vi "MyrioProject.vi"() -> ()   [LabVIEW 2018]
doc: "The myRIO Project template acquires acceleration data from the onboard accelerometer and displays the changes of acceleration values in a waveform chart."
uses:
  <vilib>/Platform/TimedLoop/XDataNode/timing_clust.ctl
  <vilib>/Platform/TimedLoop/XDataNode/nitl_modes.ctl
  <vilib>/Platform/TimedLoop/XDataNode/wakeup.ctl
  <vilib>/myRIO/Common/Instrument Driver Framework/myRIO v1.0/Encoder/typedefs/Encoder Signal Mode.ctl
  <vilib>/myRIO/Instrument Drivers/Onboard IO/PWM/typedefs/PWM Reference.ctl
  <vilib>/myRIO/Common/Instrument Driver Framework/Utilities/typedefs/myRIO Generic Hardware Reference.ctl
  <vilib>/myRIO/Common/Instrument Driver Framework/Utilities/typedefs/Hardware Version Enum.ctl
  <vilib>/myRIO/Common/Instrument Driver Framework/Utilities/typedefs/myRIO v1.0 Reference.ctl
  <vilib>/myRIO/Common/Instrument Driver Framework/Utilities/typedefs/Generic FPGA Reference.ctl
  <vilib>/myRIO/Common/Instrument Driver Framework/myRIO v1.0/PWM/typedefs/PWM Channels Enum.ctl
  <vilib>/myRIO/Instrument Drivers/Onboard IO/PWM/typedefs/PWM Configuration.ctl
  <vilib>/userdefined/High Color/nirio_resource_hc.ctl
  <vilib>/myRIO/Common/Instrument Driver Framework/myRIO v1.0/Encoder/typedefs/Encoder Configuration v1.0.ctl
  <vilib>/myRIO/Instrument Drivers/Onboard IO/Encoder/typedefs/Encoder Reference.ctl
  <vilib>/myRIO/Common/Instrument Driver Framework/myRIO v1.0/Encoder/typedefs/Encoder Channels Enum.ctl
  <vilib>/myRIO/Instrument Drivers/Onboard IO/DIO/typedefs/DIO Reference.ctl
  <vilib>/myRIO/Common/Instrument Driver Framework/myRIO v1.0/DIO/typedefs/DIO Channels List.ctl
  <vilib>/myRIO/Common/Instrument Driver Framework/myRIO v1.0/DIO/typedefs/DIO Channels Enum.ctl
  <vilib>/myRIO/Instrument Drivers/Onboard IO/AI/typedefs/AI Reference.ctl
  <vilib>/myRIO/Common/Instrument Driver Framework/myRIO v1.0/AI/typedefs/AI Channels List.ctl
  <vilib>/myRIO/Common/Instrument Driver Framework/myRIO v1.0/AI/typedefs/AI Channels Enum.ctl
  <vilib>/myRIO/Common/Instrument Driver Framework/Utilities/typedefs/Analog Scaling Constants List.ctl
  <vilib>/myRIO/Common/Instrument Driver Framework/Utilities/typedefs/Analog Scaling Constants.ctl
  <vilib>/myRIO/Common/Instrument Driver Framework/myRIO v1.0/PWM/vis/myRIO v1.1 Open PWM.vi
  <vilib>/myRIO/Common/Instrument Driver Framework/myRIO v1.0/Encoder/vis/myRIO v1.1 Open Encoder.vi
  <vilib>/myRIO/Common/Instrument Driver Framework/Utilities/vis/Is FPGA Ref Available.vi
  <vilib>/myRIO/Common/Instrument Driver Framework/myRIO v1.0/AI/vis/myRIO v1.1 Open AI.vi
  <vilib>/myRIO/Common/Instrument Driver Framework/myRIO v1.0/DIO/vis/myRIO v1.1 Open DIO.vi
  <vilib>/myRIO/Instrument Drivers/Onboard IO/PWM/vis/Set Duty Cycle and Frequency.vi
  <vilib>/myRIO/Instrument Drivers/Onboard IO/DIO/vis/Write.vi
  <vilib>/myRIO/Common/Instrument Driver Framework/Utilities/vis/Validate Channels.vi
  <vilib>/myRIO/Common/Instrument Driver Framework/myRIO v1.0/PWM/vis/myRIO v1.0 Reserve PWM.vi
  <vilib>/myRIO/Common/Instrument Driver Framework/myRIO v1.0/Encoder/vis/myRIO v1.0 Reserve Encoder.vi
  <vilib>/myRIO/Common/Instrument Driver Framework/myRIO v1.0/AI/vis/myRIO v1.0 Reserve AI.vi
  <vilib>/myRIO/Common/Instrument Driver Framework/myRIO v1.0/DIO/vis/myRIO v1.0 Reserve DIO.vi
  <vilib>/myRIO/Common/Instrument Driver Framework/myRIO v1.0/Encoder/vis/myRIO v1.0 Close Encoder.vi
  <vilib>/myRIO/Common/Instrument Driver Framework/myRIO v1.0/PWM/vis/myRIO v1.0 Close PWM.vi
  <vilib>/myRIO/Common/Instrument Driver Framework/myRIO v1.0/PWM/vis/myRIO v1.0 Build MUX Configuration PWM.vi
  <vilib>/myRIO/Common/Instrument Driver Framework/myRIO v1.0/Resource Manager/vis/myRIO v1.0 Reserve Channel List.vi
  <vilib>/myRIO/Common/Instrument Driver Framework/myRIO v1.0/Encoder/vis/myRIO v1.0 Build MUX Configuration Encoder.vi
  <vilib>/myRIO/Common/Instrument Driver Framework/myRIO v1.0/AI/vis/myRIO v1.0 Build MUX Configuration AI.vi
  <vilib>/myRIO/Common/Instrument Driver Framework/myRIO v1.0/DIO/vis/myRIO v1.0 Build MUX Configuration DIO.vi
  <vilib>/myRIO/Common/Instrument Driver Framework/myRIO v1.0/Encoder/vis/myRIO v1.0 Unreserve Encoder.vi
  <vilib>/myRIO/Common/Instrument Driver Framework/myRIO v1.0/PWM/vis/myRIO v1.0 Unreserve PWM.vi
  <vilib>/myRIO/Common/Instrument Driver Framework/myRIO v1.0/Resource Manager/vis/myRIO v1.0 Create Configuration List.vi
  <vilib>/myRIO/Common/Instrument Driver Framework/myRIO v1.0/Resource Manager/vis/myRIO v1.0 Reserve Channel.vi
  <vilib>/myRIO/Common/Instrument Driver Framework/myRIO v1.0/Resource Manager/vis/myRIO v1.0 Unreserve Channel.vi
  <vilib>/myRIO/Common/Instrument Driver Framework/myRIO v1.0/Resource Manager/vis/myRIO v1.0 Unreserve Channel List.vi
  <vilib>/myRIO/Common/Instrument Driver Framework/myRIO v1.0/Resource Manager/vis/myRIO v1.0 Build Mutex Name.vi
  <vilib>/Utility/VariantDataType/GetNumericInfo.vi
  <vilib>/Utility/error.llb/Error Cluster From Error Code.vi
  <vilib>/myRIO/Common/Instrument Driver Framework/myRIO v1.0/myRIO v1.1 Open.vi
  <vilib>/myRIO/Common/Instrument Driver Framework/Utilities/vis/IO Manager.vi
  <vilib>/myRIO/Common/Instrument Driver Framework/Utilities/vis/Configuration Manager.vi
  <vilib>/myRIO/Common/Instrument Driver Framework/myRIO v1.0/Resource Manager/vis/myRIO v1.0 Configure IO.vi
  <vilib>/myRIO/Common/Instrument Driver Framework/myRIO v1.0/myRIO v1.0 Close.vi
  <vilib>/myRIO/Common/Instrument Driver Framework/myRIO v1.0/PWM/vis/myRIO v1.0 Write PWM.vi
  <vilib>/myRIO/Common/Instrument Driver Framework/myRIO v1.0/Encoder/vis/myRIO v1.0 Configure Encoder.vi
  <vilib>/myRIO/Common/Instrument Driver Framework/myRIO v1.0/Encoder/vis/myRIO v1.0 Enable Encoder.vi
  <vilib>/myRIO/Common/Instrument Driver Framework/myRIO v1.0/DIO/vis/myRIO v1.0 Read DIO.vi
  <vilib>/myRIO/Common/Instrument Driver Framework/myRIO v1.0/AI/vis/myRIO v1.0 Get Scaling Constants AI.vi
  <vilib>/myRIO/Common/Instrument Driver Framework/myRIO v1.0/AI/vis/myRIO v1.0 Read AI.vi
  <vilib>/myRIO/Common/Instrument Driver Framework/myRIO v1.0/Encoder/vis/myRIO v1.0 Read Encoder.vi
  <vilib>/myRIO/Common/Instrument Driver Framework/myRIO v1.0/DIO/vis/myRIO v1.0 Write DIO.vi
  <vilib>/myRIO/Common/Instrument Driver Framework/myRIO v1.0/Encoder/vis/myRIO v1.0 Shutdown Encoder.vi
  <vilib>/myRIO/Common/Instrument Driver Framework/myRIO v1.0/PWM/vis/myRIO v1.0 Shutdown PWM.vi
  <vilib>/platform/TimedLoop/XDataNode/XDataNode.xnode
  <vilib>/myRIO/Instrument Drivers/Onboard IO/PWM/vis/myRIO PWM Open.xnode
  <vilib>/myRIO/Instrument Drivers/Onboard IO/Encoder/vis/myRIO Encoder Open.xnode
  <vilib>/myRIO/Express VI/Onboard IO/PWM/PWM Express VI.xnode
  <vilib>/myRIO/Express VI/Onboard Devices/Button/Button Express VI.xnode
  <vilib>/myRIO/Instrument Drivers/Onboard IO/DIO/vis/myRIO DIO Open.xnode
  <vilib>/myRIO/Express VI/Onboard IO/AI/AI Express VI.xnode
  <vilib>/myRIO/Instrument Drivers/Onboard IO/AI/vis/myRIO AI Open.xnode
  <vilib>/myRIO/Express VI/Onboard IO/DO/DO Express VI.xnode
  <vilib>/Platform/TimedLoop/XDataNode/XDNodeRunTimeDep.lvlib
  <vilib>/myRIO/Instrument Drivers/Onboard IO/Encoder/Encoder.lvlib
  <vilib>/myRIO/Instrument Drivers/Onboard IO/PWM/PWM.lvlib
  <vilib>/myRIO/Instrument Drivers/Onboard IO/DIO/DIO.lvlib
  <vilib>/myRIO/Instrument Drivers/Onboard IO/AI/AI.lvlib
panel:
  out "Waveform Chart":dbl(graph)
  out "Numeric Control":dbl
  out "data":dbl
  out "Double 2":dbl
  out "Double":dbl
  out "sensor2 (A/AI2 (Pin 7))":dbl
  out "sensor1":dbl
  out "stallRojo (A/AI0 (Pin 3))":dbl
  out "stallBlanco (A/AI1 (Pin 5))":dbl
  in  "MANUAL 2":bool
  in  "Stop Button":bool
  in  "Start":bool
  out "element":dbl
  out "element 2":dbl
  out "subarray 2":dbl[][](array[numeric])
  out "subarray":dbl[][](array[numeric])
  out "vectores":dbl[][][](array[numeric])
  in  "saturacion":dbl=0.3
  in  "Duty Cycle 2":dbl(slide)=0.5 scale=0.05..0.1
  in  "Duty Cycle":dbl(slide)=0.5 scale=0.05..0.1
  in  "Reset Counter 2":bool
  in  "Reset Counter":bool
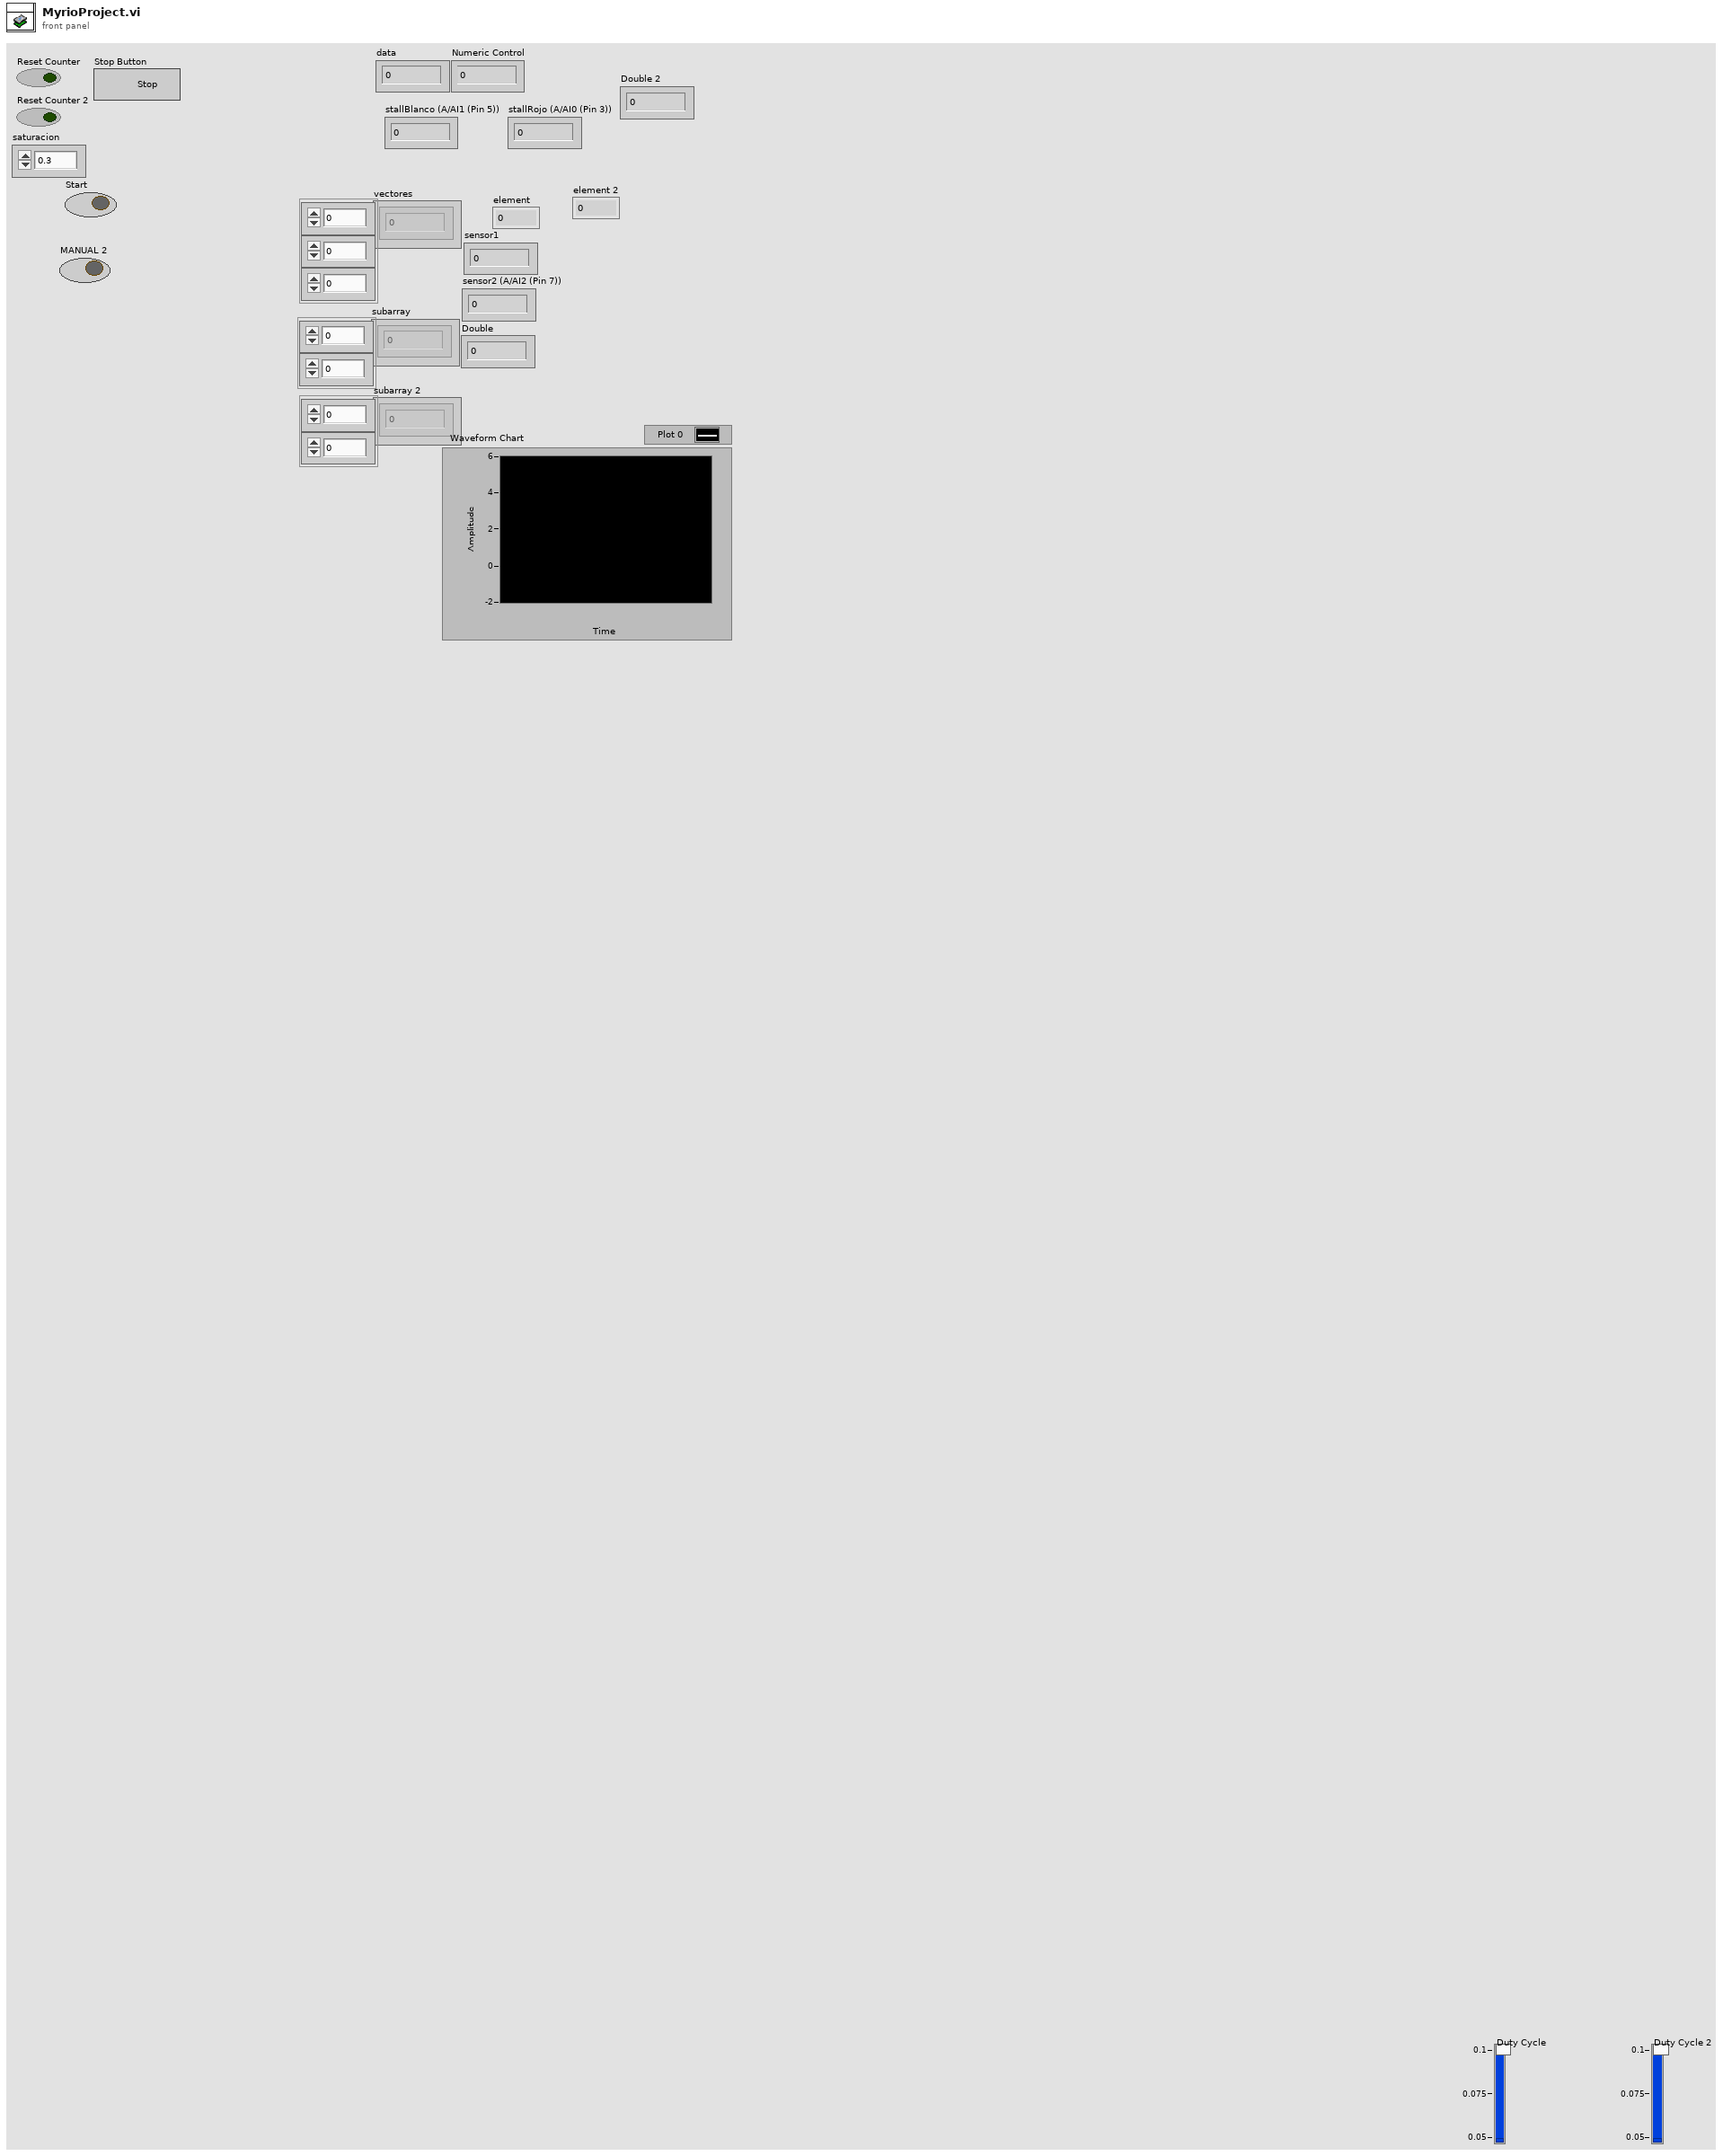
[diagram p1: front panel]
types:
  T1 = enum16{"normal", "grande-Sensor", "grande home", "peque-sensor", "peque- home", "peque-reset"}
  T2 = typedef "Encoder Signal Mode.ctl" = enum16{"Quadrature phase signal", "Step and direction signal"}
  T3 = typedef "PWM.lvlib/PWM Reference.ctl" = cluster{"myRIO Reference":T4, "PWM Channels Enum":T8, "PWM Configuration":T9}
  T4 = typedef "myRIO Generic Hardware Reference.ctl" = cluster{"myRIO Model":T5, "myRIO Hardware Reference":T6}
  T5 = typedef "Hardware Version Enum.ctl" = enum16{"Unknown", "myRIO-1900", "myRIO-1950", "roboRIO", "NI ELVIS RIO CM", "ELVIS III"}
  T6 = typedef "myRIO v1.0 Reference.ctl" = cluster{"Generic FPGA Reference":T7, "Allow multiple opens":bool}
  T7 = typedef "Generic FPGA Reference.ctl" = refnum<k20>
  T8 = typedef "PWM Channels Enum.ctl" = enum16{"Not Connected", "C/PWM0", "C/PWM1", "A/PWM0", "A/PWM1", "A/PWM2", "A/PWM3", "A/PWM4", "A/PWM5", "A/PWM6", "A/PWM7", "A/PWM8", "A/PWM9", "A/PWM10", "A/PWM11", "A/PWM12", "A/PWM13", "A/PWM14", "A/PWM15", "A/PWM16", "A/PWM17", "A/PWM18", "A/PWM19", "B/PWM0", "B/PWM1", "B/PWM2", "B/PWM3", "B/PWM4", "B/PWM5", "B/PWM6", "B/PWM7", "B/PWM8", "B/PWM9", "B/PWM10", "B/PWM11", "B/PWM12", "B/PWM13", "B/PWM14", "B/PWM15", "B/PWM16", "B/PWM17", "B/PWM18", "B/PWM19", "PWM/PWM0", "PWM/PWM1", "PWM/PWM2", "PWM/PWM3", "PWM/PWM4", "PWM/PWM5", "PWM/PWM6", "PWM/PWM7", "PWM/PWM8", "PWM/PWM9"}
  T9 = typedef "PWM.lvlib/PWM Configuration.ctl" = cluster{"Frequency":dbl, "Duty Cycle":dbl}
  T10 = typedef "Encoder.lvlib/Encoder Reference.ctl" = cluster{"myRIO Reference":T4, "Encoder Channels Enum":T11}
  T11 = typedef "Encoder Channels Enum.ctl" = enum16{"Not Connected", "C/ENC0", "C/ENC1", "A/ENC", "A/ENC0", "A/ENC1", "A/ENC2", "A/ENC3", "A/ENC4", "A/ENC5", "A/ENC6", "A/ENC7", "A/ENC8", "A/ENC9", "B/ENC", "B/ENC0", "B/ENC1", "B/ENC2", "B/ENC3", "B/ENC4", "B/ENC5", "B/ENC6", "B/ENC7", "B/ENC8", "B/ENC9", "DIO/ENC0", "DIO/ENC1", "DIO/ENC2", "DIO/ENC3", "DIO/ENC4"}
  T12 = typedef "XDNodeRunTimeDep.lvlib/timing_clust.ctl" = cluster{"Expected End [f-1]":u64, "Actual End [f-1]":u64, "Finished Late? [f-1]":bool, "Expected End [i-1]":u64, "Actual End [i-1]":u64, "Finished Late? [i-1]":bool, "Expected Start [i]":u64, "Actual Start [i]":u64, "Expected Start [f]":u64, "Actual Start [f]":u64, "Source Name":string, "Structure Name":string, "Period":i64, "Deadline":i64, "Offset":i64, "Start":i64, "Priority":i32, "Timeout":i32, "Mode":T13, "Wakeup Reason":T14, "Error":errorcluster, "Source Type":string, "Secondary Source Type":string, "Global End Time":u64, "Global Start Time":u64, "Frame Duration":u64, "Iteration Duration":u64, "Assigned CPU":i32, "I/O Scan Engine Mode":u32}
  T13 = typedef "XDNodeRunTimeDep.lvlib/nitl_modes.ctl" = enum32{"No Change", "Process missed periods, maintain original phase", "Discard missed periods, maintain original phase", "Process missed periods, ignore original phase", "Discard missed periods, ignore original phase"}
  T14 = typedef "XDNodeRunTimeDep.lvlib/wakeup.ctl" = enum32{"Normal", "Aborted", "Asynchronous wakeup", "Timing source error", "Timed loop error", "Timeout"}
  T15 = typedef "nirio_resource_hc.ctl" = tag
  T16 = typedef "AI.lvlib/AI Reference.ctl" = cluster{"myRIO Reference":T4, "AI Channels List":T17, "AI Scaling Constants List":T19}
  T17 = typedef "AI Channels List.ctl" = T18[]
  T18 = typedef "AI Channels Enum.ctl" = enum16{"Not Connected", "AudioIn/Left", "AudioIn/Right", "C/AI0", "C/AI1", "A/AI0", "A/AI1", "A/AI2", "A/AI3", "A/AI4", "A/AI5", "A/AI6", "A/AI7", "B/AI0", "B/AI1", "B/AI2", "B/AI3", "B/AI4", "B/AI5", "B/AI6", "B/AI7", "AI/AI0", "AI/AI1", "AI/AI2", "AI/AI3", "A/AI0 (DIFF)", "A/AI1 (DIFF)", "A/AI2 (DIFF)", "A/AI3 (DIFF)", "B/AI0 (DIFF)", "B/AI1 (DIFF)", "B/AI2 (DIFF)", "B/AI3 (DIFF)"}
  T19 = typedef "Analog Scaling Constants List.ctl" = T20[]
  T20 = typedef "Analog Scaling Constants.ctl" = cluster{"LSB Weight (Volts)":dbl, "Offset (Volts)":dbl, "Signed?":bool}
  T21 = typedef "DIO.lvlib/DIO Reference.ctl" = cluster{"myRIO Reference":T4, "DIO Channels List":T22}
  T22 = typedef "DIO Channels List.ctl" = T23[]
  T23 = typedef "DIO Channels Enum.ctl" = enum16{"Not Connected", "C/DIO0", "C/DIO1", "C/DIO2", "C/DIO3", "C/DIO4", "C/DIO5", "C/DIO6", "C/DIO7", "A/DIO0", "A/DIO1", "A/DIO2", "A/DIO3", "A/DIO4", "A/DIO5", "A/DIO6", "A/DIO7", "A/DIO8", "A/DIO9", "A/DIO10", "A/DIO11", "A/DIO12", "A/DIO13", "A/DIO14", "A/DIO15", "A/DIO16", "A/DIO17", "A/DIO18", "A/DIO19", "B/DIO0", "B/DIO1", "B/DIO2", "B/DIO3", "B/DIO4", "B/DIO5", "B/DIO6", "B/DIO7", "B/DIO8", "B/DIO9", "B/DIO10", "B/DIO11", "B/DIO12", "B/DIO13", "B/DIO14", "B/DIO15", "B/DIO16", "B/DIO17", "B/DIO18", "B/DIO19", "LED0", "LED1", "LED2", "LED3", "Button0", "DIO/DIO0", "DIO/DIO1", "DIO/DIO2", "DIO/DIO3", "DIO/DIO4", "DIO/DIO5", "DIO/DIO6", "DIO/DIO7", "DIO/DIO8", "DIO/DIO9", "SPI/CS0", "SPI/CS1", "SPI/CS2", "SPI/CS3", "LED RADIO (Green)", "LED RADIO (Red)", "LED COMM (Green)", "LED COMM (Red)", "LED MODE (Green)", "LED MODE (Red)"}
  T24 = cluster{dbl, dbl, "Counter Value":i32, "seconds since 1Jan1904":timestamp, dbl, dbl, dbl}
  T25 = cluster{"Double":dbl, "dbl Scaled Value":dbl, "Output":dbl, "seconds since 1Jan1904":timestamp, dbl, dbl, dbl}
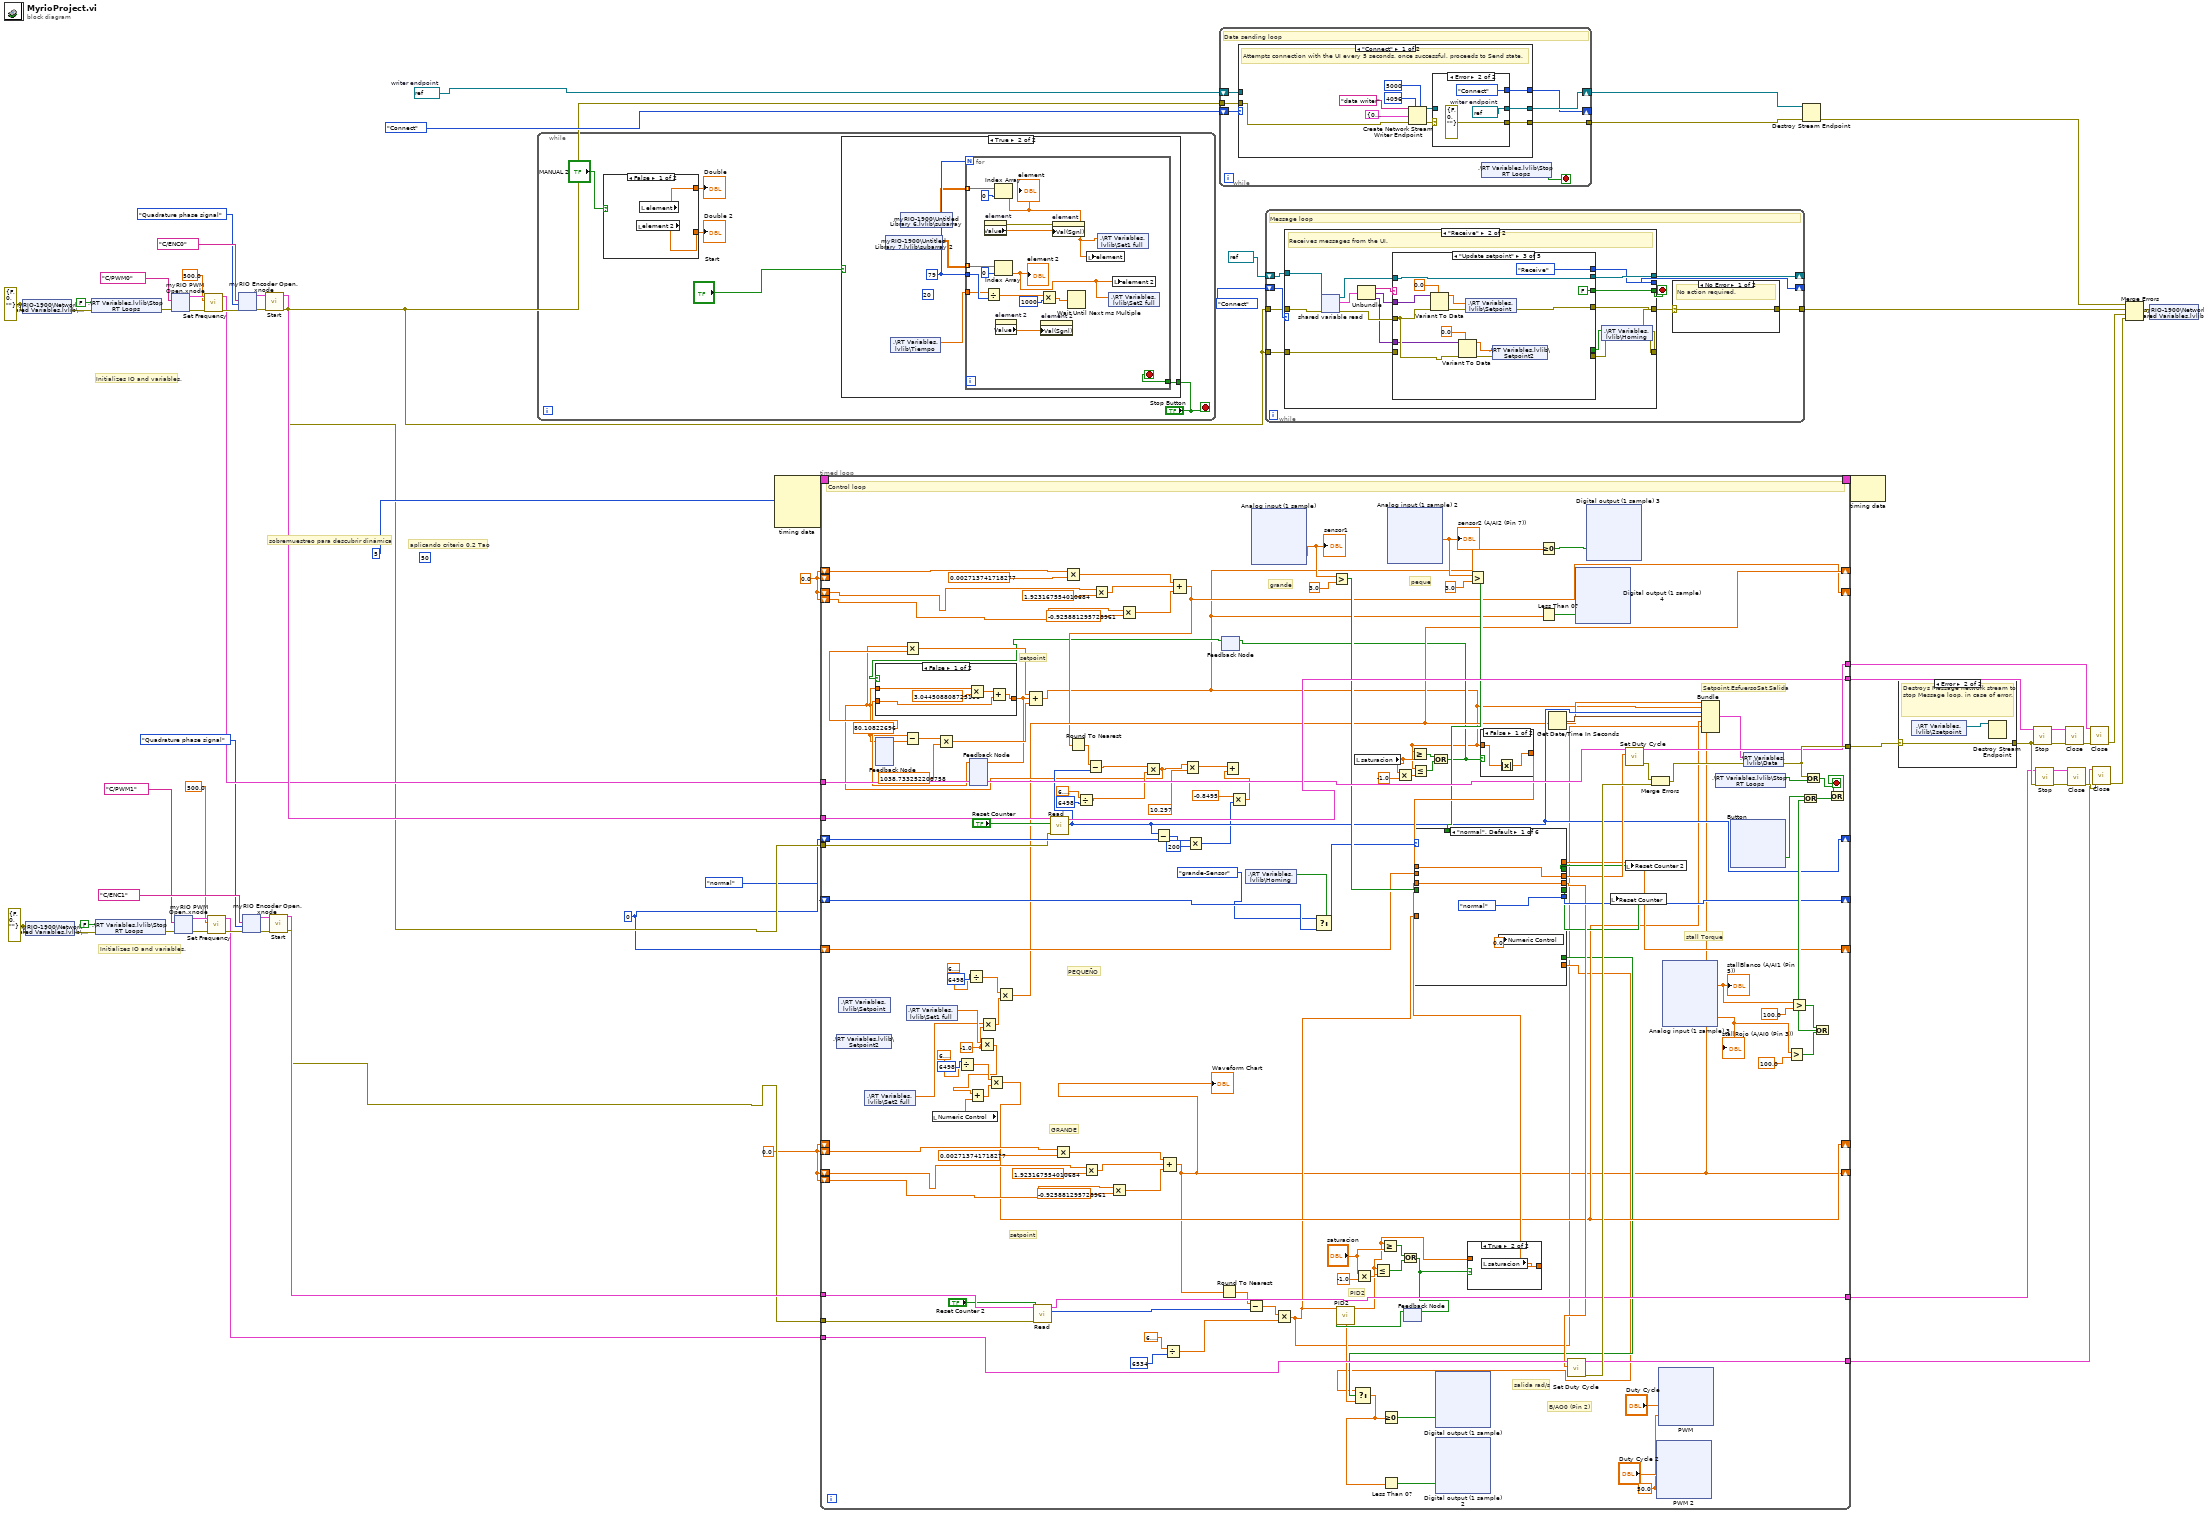
[diagram p0: block diagram]
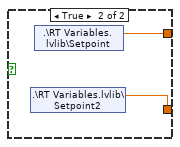
[diagram p2: hidden frame]
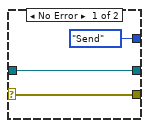
[diagram p5: hidden frame]
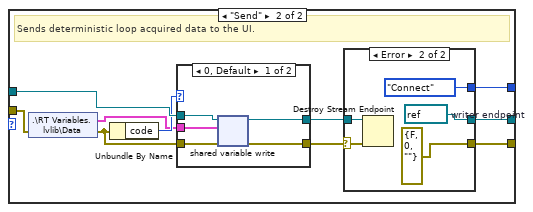
[diagram p6: hidden frame]
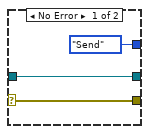
[diagram p7: hidden frame]
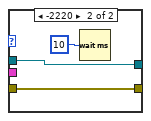
[diagram p8: hidden frame]
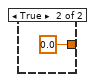
[diagram p9: hidden frame]
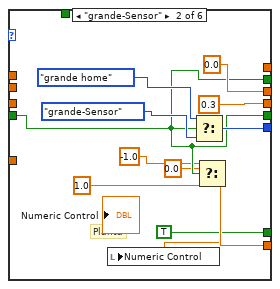
[diagram p10: hidden frame]
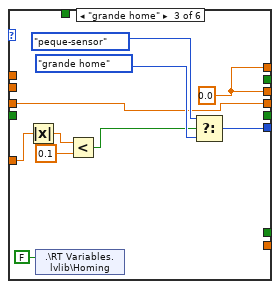
[diagram p11: hidden frame]
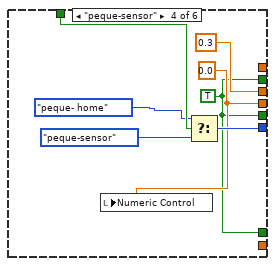
[diagram p12: hidden frame]
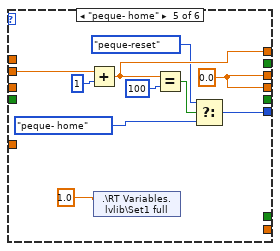
[diagram p13: hidden frame]
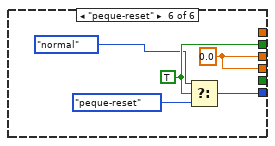
[diagram p14: hidden frame]
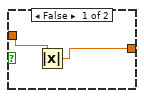
[diagram p15: hidden frame]
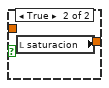
[diagram p16: hidden frame]
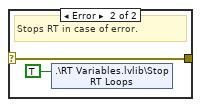
[diagram p17: hidden frame]
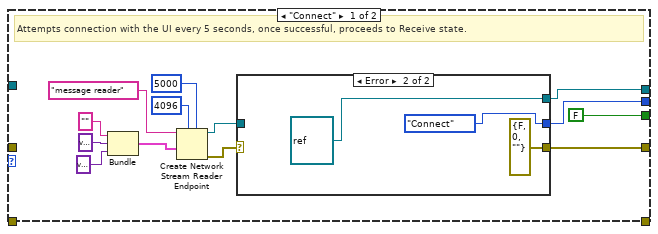
[diagram p18: hidden frame]
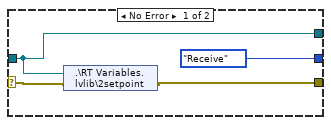
[diagram p19: hidden frame]
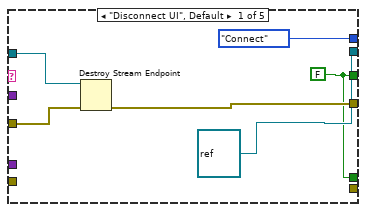
[diagram p20: hidden frame]
diagram:
  w2 = 0.0
  w3 = 0.0
  w4 = 0
  (unwired) 50
  w16 = refnum<k21> refnum  # writer endpoint
  w29 = errorcluster {"status"=FALSE, "code"=0, "source"=""} ("error IO")
  w51 = errorcluster {"status"=FALSE, "code"=0, "source"=""} ("error IO")
  # "aplicando criterio 0.2 Tao"
  # "sobremuestreo para descubrir dinámica"
  # "Initializes IO and variables."
  # "Initializes IO and variables."
  n1 = shared-variable "myRIO-1900\\Network Shared Variables.lvlib\\error IO"(w51, error in=w51) -> (error out=w52:errorcluster)
  n2 = shared-variable "myRIO-1900\\Network Shared Variables.lvlib\\error IO"(w29, error in=w29) -> (error out=w30:errorcluster)
  n3 = shared-variable ".\\RT Variables.lvlib\\Stop RT Loops"(FALSE ("Stop RT Loops"), error in=w52) -> (error out=w39:errorcluster)
  n4 = shared-variable ".\\RT Variables.lvlib\\Stop RT Loops"(FALSE ("Stop RT Loops"), error in=w30) -> (error out=w22:errorcluster)
  n5 = xnode "myRIO PWM Open.xnode"("error in (no error)"=w39, "Channel Name"=tag "C/PWM0") -> ("error out"=w41:errorcluster, "PWM Ref Out"=w40:T3)  [unwired: 1 in]
  n6 = xnode "myRIO PWM Open.xnode"("error in (no error)"=w22, "Channel Name"=tag "C/PWM1") -> ("error out"=w24:errorcluster, "PWM Ref Out"=w23:T3)  [unwired: 1 in]
  n7 = call <vilib>:"Set Frequency.vi"("error in (no error)"=w41, "Frequency [Hz]"=500.0, "PWM Ref In"=w40) -> ("error out"=w38:errorcluster, "PWM Ref Out"=w35:T3)  [unwired: 6 in]
  n8 = call <vilib>:"Set Frequency.vi"("error in (no error)"=w24, "Frequency [Hz]"=500.0, "PWM Ref In"=w23) -> ("error out"=w21:errorcluster, "PWM Ref Out"=w17:T3)  [unwired: 6 in]
  n9 = xnode "myRIO Encoder Open.xnode"("error in (no error)"=w38, "Channel Name"=tag "C/ENC0", "Encoder Signal Mode"=Encoder_Signal_Mode."Quadrature phase signal") -> ("error out"=w48:errorcluster, "Encoder Ref Out"=w47:T10)  [unwired: 2 in]
  n10 = xnode "myRIO Encoder Open.xnode"("error in (no error)"=w21, "Channel Name"=tag "C/ENC1", "Encoder Signal Mode"=Encoder_Signal_Mode."Quadrature phase signal") -> ("error out"=w27:errorcluster, "Encoder Ref Out"=w26:T10)  [unwired: 2 in]
  n11 = call <vilib>:"Start.vi"("error in (no error)"=w48, "Encoder Ref In"=w47) -> ("error out"=w6:errorcluster, "Encoder Ref Out"=w45:T10)  [unwired: 8 in]
  n12 = call <vilib>:"Start.vi"("error in (no error)"=w27, "Encoder Ref In"=w26) -> ("error out"=w5:errorcluster, "Encoder Ref Out"=w18:T10)  [unwired: 8 in]
  n13 = while {
    stop <- "Stop Button" stop-if-true
    n14 = case shown="False" "MANUAL 2" {
      tunnel: [w69 w71] -> w63
      tunnel: [w68 w70] -> w64
      frame False {
        n15 = local read "element 2"() -> (w69:dbl)
        n16 = local read "element"() -> (w68:dbl)
      }
      frame True {
        n17 = shared-variable ".\\RT Variables.lvlib\\Setpoint2"() -> (w71:dbl)  [unwired: 1 in, 1 out]
        n18 = shared-variable ".\\RT Variables.lvlib\\Setpoint"() -> (w70:dbl)  [unwired: 1 in, 1 out]
      }
    }
    "Double" <- w64
    "Double 2" <- w63
    n19 = case shown="True" "Start" {
      tunnel: "Stop Button" -> [_ w73]
      frame False {
      }
      frame True {
        (unwired) 20
        w76 = 79
        n20 = shared-variable "myRIO-1900\\Untitled Library 7.lvlib\\subarray 2"() -> (w74:dbl[][])  [unwired: 1 in, 1 out]
        n21 = shared-variable ".\\RT Variables.lvlib\\Tiempo"() -> (w72:dbl)  [unwired: 1 in, 1 out]
        n22 = shared-variable "myRIO-1900\\Untitled Library 6.lvlib\\subarray"() -> (w75:dbl[][])  [unwired: 1 in, 1 out]
        n23 = for {
          N: w76 -> [_]
          tunnel: w76 -> [w89]
          tunnel: w75 -> [w88] mode=indexing
          tunnel: w72 -> [w86]
          tunnel: w74 -> [w84] mode=indexing
          tunnel: w73 -> [w79]
          stop <- w79 stop-if-true
          n24 = property on="element" class="DigNum (strict)"() -> (error out=w82:errorcluster, "Value"=w83:dbl)  [unwired: 2 in, 1 out]
          n25 = Divide(x=w86, y=w89) -> (x/y=w91:dbl)
          n26 = Index Array(array=w88, index=0) -> (element=w78:dbl)
          "element" <- w78
          n27 = Index Array(array=w84, index=0) -> (element=w77:dbl)
          "element 2" <- w77
          n28 = property on="element 2" class="DigNum (strict)"() -> ("Value"=w81:dbl)  [unwired: 2 in, 2 out]
          n29 = Multiply(x=w91, y=1000) -> (x*y=w80:dbl)
          n30 = property on="element 2" class="DigNum (strict)"("Val(Sgnl)"=w81) -> ()  [unwired: 2 in, 2 out]
          n31 = property on="element" class="DigNum (strict)"(error in=w82, "Val(Sgnl)"=w83) -> ()  [unwired: 1 in, 2 out]
          n32 = Wait Until Next ms Multiple(millisecond multiple=w80) -> ()  [unwired: 1 out]
          n33 = local write "element"(w78) -> ()
          n34 = shared-variable ".\\RT Variables.lvlib\\Set1 full"(w78) -> ()  [unwired: 1 in, 1 out]
          n35 = shared-variable ".\\RT Variables.lvlib\\Set2 full"(w77) -> ()  [unwired: 1 in, 1 out]
          n36 = local write "element 2"(w77) -> ()
        }
      }
    }
  }
  n37 = node-c288(i64 5 ("Period")) -> (w62:T12)  [unwired: 3 in]
  n38 = timed-loop {
    timing: w62 -> [_]
    timing-out: [_] -> w61
    tunnel: [w229] -> w50
    tunnel: w45 -> [w195]
    tunnel: [w194] -> w42
    tunnel: w35 -> [w183]
    tunnel: [w228] -> w34
    tunnel: w18 -> [w225]
    tunnel: w17 -> [w224]
    tunnel: [w220] -> w11
    tunnel: [w219] -> w10
    shift-right: [w145] -> _
    shift-left: w3 -> [_]
    shift-left: w3 -> [w206]
    shift-right: [w97] -> _
    shift-left: w3 -> [w205]
    shift-left: w3 -> [w204]
    shift-right: [w180] -> _
    shift-left: T1."normal" ("Enum") -> [w179]
    shift-right: [w174] -> _
    shift-left: w4 -> [w173]
    shift-right: [w162] -> _
    shift-left: w4 -> [w163]
    tunnel: w5 -> [w157]
    tunnel: w6 -> [w156]
    shift-right: [w112] -> _
    shift-left: w2 -> [w116]
    shift-right: [w111] -> _
    shift-left: w2 -> [w115]
    shift-left: w2 -> [w114]
    shift-left: w2 -> [_]
    stop <- w217 stop-if-true
    w92 = -1.0 ("y")
    w159 = 50.0 ("Frequency [Hz]")
    # "setpoint"
    # "PEQUEÑO"
    # "peque"
    # "grande"
    # "stall Torque"
    # "Setpoint,EsfuersoSat,Salida"
    # "setpoint"
    # "PID2"
    # "GRANDE"
    # "salida rad/s"
    # "B/AO0 (Pin 2)"
    # "Control loop"
    n39 = shared-variable ".\\RT Variables.lvlib\\Setpoint2"() -> ()  [unwired: 1 in, 2 out]
    n40 = shared-variable ".\\RT Variables.lvlib\\Setpoint"() -> ()  [unwired: 1 in, 2 out]
    n41 = shared-variable ".\\RT Variables.lvlib\\Set2 full"() -> (w93:dbl)  [unwired: 1 in, 1 out]
    n42 = feedback #1() -> (w124:dbl)  [unwired: 1 in]
    n43 = shared-variable ".\\RT Variables.lvlib\\Set1 full"() -> (w96:dbl)  [unwired: 1 in, 1 out]
    n44 = local read "Numeric Control"() -> (w101:dbl)
    n45 = Divide(x=6498, y=6.283185307179586) -> (x/y=w146:dbl)
    n46 = Divide(x=6498, y=6.283185307179586) -> (x/y=w149:dbl)
    n47 = feedback #2() -> (w118:dbl)  [unwired: 1 in]
    n48 = Multiply(x=w96, y=w92) -> (x*y=w95:dbl)
    n49 = Add(x=w95, y=w101) -> (x+y=w98:dbl)
    n50 = Multiply(x=w93, y=w92) -> (x*y=w94:dbl)
    n51 = Multiply(x=w146, y=w98) -> (x*y=w145:dbl)
    n52 = Multiply(x=w149, y=w94) -> (x*y=w112:dbl)
    n53 = call <vilib>:"Read.vi"("error in (no error)"=w157, "Reset Counter"="Reset Counter 2", "Encoder Ref In"=w225) -> ("Counter Value"=w200:i32, "Encoder Ref Out"=w220:T10)  [unwired: 4 in, 3 out]
    n54 = call <vilib>:"Read.vi"("error in (no error)"=w156, "Reset Counter"="Reset Counter", "Encoder Ref In"=w195) -> ("Counter Value"=w162:i32, "Encoder Ref Out"=w194:T10)  [unwired: 4 in, 3 out]
    n55 = Multiply(x=w206, y=0.002713741718277) -> (x*y=w208:dbl)
    n56 = Multiply(x=w116, y=0.002713741718277) -> (x*y=w129:dbl)
    n57 = Divide(x=6.283185307179586, y=6498) -> (x/y=w165:dbl)
    n58 = Multiply(x=w205, y=1.923167554010684) -> (x*y=w209:dbl)
    n59 = Multiply(x=w115, y=1.923167554010684) -> (x*y=w128:dbl)
    n60 = Multiply(x=w204, y=-0.925881295728961) -> (x*y=w207:dbl)
    n61 = Multiply(x=w114, y=-0.925881295728961) -> (x*y=w130:dbl)
    n62 = Subtract(x=w162, y=w163) -> (x-y=w134:i32)
    n63 = Compound Arithmetic op=ADD(w208, w209, w207) -> (w97:dbl)
    "Waveform Chart" <- w97
    n64 = Divide(x=6.283185307179586, y=6534) -> (x/y=w199:dbl)
    n65 = Compound Arithmetic op=ADD(w129, w128, w130) -> (w111:dbl)
    n66 = Round To Nearest(number=w111) -> (nearest integer value=w193:dbl)
    n67 = Subtract(x=w193, y=w162) -> (x-y=w164:dbl)
    n68 = Multiply(x=w164, y=w165) -> (x*y=w113:dbl)
    n69 = feedback-in #1(w113) -> ()
    n70 = Multiply(x=w113, y=80.10822696) -> (x*y=w122:dbl)
    n71 = Subtract(x=w113, y=w124) -> (x-y=w121:dbl)
    n72 = Multiply(x=w121, y=1038.733252208758) -> (x*y=w120:dbl)
    n73 = Multiply(x=w113, y=10.297) -> (x*y=w167:dbl)
    n74 = Multiply(x=w134, y=200) -> (x*y=w132:i32)
    n75 = Round To Nearest(number=w97) -> (nearest integer value=w198:dbl)
    n76 = feedback #3() -> (w109:bool)  [unwired: 1 in]
    n77 = case shown="False" w109 {
      tunnel: w113 -> [w235 _]
      tunnel: [w233 0.0 ("x")] -> w117
      tunnel: w118 -> [w232 _]
      frame False {
        n78 = Multiply(x=w235, y=3.044508808725106 ("x")) -> (x*y=w234:dbl)
        n79 = Add(x=w234, y=w232) -> (x+y=w233:dbl)
      }
      frame True {
      }
    }
    n80 = feedback-in #2(w117) -> ()
    n81 = Compound Arithmetic op=ADD(w122, w117, w120) -> (w108:dbl)
    n82 = Multiply(x=-0.8495, y=w132) -> (x*y=w166:dbl)
    n83 = Add(x=w167, y=w166) -> ()  [unwired: 1 out]
    n84 = shared-variable ".\\RT Variables.lvlib\\Homing"() -> (w184:bool)  [unwired: 1 in, 1 out]
    n85 = Subtract(x=w198, y=w200) -> (x-y=w100:dbl)
    n86 = xnode "Analog input (1 sample)"() -> ("A/AI3 (Pin 9)"=w153:dbl)  [unwired: 1 in, 1 out]
    "sensor1" <- w153
    n87 = Multiply(x=w100, y=w199) -> (x*y=w99:dbl)
    n88 = Select(t=T1."grande-Sensor" ("Enum"), s=w184, f=w179) -> (s? t:f=w106:T1)
    n89 = Greater?(x=w153, y=3.0) -> (0:w178:bool)
    n90 = local read "saturacion"() -> (w140:dbl)
    n91 = Multiply(x="saturacion", y=-1.0) -> (x*y=w139:dbl)
    n92 = xnode "Analog input (1 sample) 2"() -> ("sensor2 (A/AI2 (Pin 7))"=w152:dbl)  [unwired: 1 in, 1 out]
    "sensor2 (A/AI2 (Pin 7))" <- w152
    n93 = Multiply(x=w140, y=-1.0) -> (x*y=w142:dbl)
    n94 = feedback #4() -> (w203:bool)  [unwired: 1 in]
    n95 = call "PID2.vi"("Boolean"=w203, "Numeric in"=w99) -> ("Numeric out"=w103:dbl)  [unwired: 9 in]
    n96 = Less Or Equal?(x=w103, y=w139) -> (x <= y?=w213:bool)
    n97 = Greater Or Equal?(x=w103, y="saturacion") -> (x >= y?=w214:bool)
    n98 = Or(x=w214, y=w213) -> (x .or. y?=w202:bool)
    n99 = feedback-in #4(w202) -> ()
    n100 = Greater Or Equal?(x=w108, y=w140) -> (x >= y?=w216:bool)
    n101 = Less Or Equal?(x=w108, y=w142) -> (x <= y?=w215:bool)
    n102 = Or(x=w216, y=w215) -> (x .or. y?=w110:bool)
    n103 = feedback-in #3(w110) -> ()
    n104 = case shown="True" w202 {
      tunnel: [w607 w609] -> w177
      tunnel: w103 -> [w608 _]
      frame False {
        n105 = Absolute Value(x=w608) -> (abs(x)=w607:dbl)
      }
      frame True {
        n106 = local read "saturacion"() -> (w609:dbl)
      }
    }
    n107 = Greater?(x=w152, y=3.0) -> (0:w175:bool)
    n108 = case shown="False" w110 {
      tunnel: [w610 w612] -> w182
      tunnel: w108 -> [w611 _]
      frame False {
        n109 = Absolute Value(x=w611) -> (abs(x)=w610:dbl)
      }
      frame True {
        n110 = local read "saturacion"() -> (w612:dbl)
      }
    }
    n111 = case shown="\"normal\", Default" w106 {
      tunnel: w182 -> [w311 _ _ _ _ _]
      tunnel: [w311 0.0 ("f") w329 0.3 ("f") w340 w354] -> w181
      tunnel: [T1."normal" ("Enum") w321 w332 w337 w346 w352] -> w180
      tunnel: w178 -> [_ w315 _ _ _ _]
      tunnel: w177 -> [w310 _ w328 _ _ _]
      tunnel: [w310 0.3 ("f") w328 w334 w340 w354] -> w176
      tunnel: w175 -> [_ _ _ w338 _ _]
      tunnel: [_ _ w329 _ w345 _] -> w174
      tunnel: w173 -> [_ _ _ _ w344 _]
      tunnel: [_ w315 _ w333 _ _] -> w171
      tunnel: [_ w315 _ w333 _ w351] -> w169
      tunnel: [_ 1.0 _ _ _ _] -> w102
      tunnel: [_ TRUE _ w333 _ _] -> w104
      tunnel: w99 -> [_ _ w327 _ _ _]
      frame "normal", Default {
        n112 = local write "Numeric Control"(0.0) -> ()
      }
      frame "grande-Sensor" {
        # "Planta"
        n113 = Select(t=T1."grande home" ("Enum"), s=w315, f=T1."grande-Sensor" ("Enum")) -> (s? t:f=w321:T1)
        n114 = Select(t=-1.0, s=w315, f=0.0) -> (s? t:f=w312:dbl)
        n115 = local write "Numeric Control"(w312) -> ()
      }
      frame "grande home" {
        w329 = 0.0
        n116 = Absolute Value(x=w327) -> (abs(x)=w326:dbl)
        n117 = shared-variable ".\\RT Variables.lvlib\\Homing"(FALSE ("Homing")) -> ()  [unwired: 1 in, 1 out]
        n118 = Less?(x=w326, y=0.1) -> (x < y?=w324:bool)
        n119 = Select(t=T1."peque-sensor" ("Enum"), s=w324, f=T1."grande home" ("Enum")) -> (s? t:f=w332:T1)
      }
      frame "peque-sensor" {
        w333 = TRUE
        w334 = 0.0 ("f")
        n120 = local write "Numeric Control"(w334) -> ()
        n121 = Select(t=T1."peque- home" ("Enum"), s=w338, f=T1."peque-sensor" ("Enum")) -> (s? t:f=w337:T1)
      }
      frame "peque- home" {
        w340 = 0.0 ("f")
        n122 = Add(x=w344, y=1) -> (x+y=w345:dbl)
        n123 = shared-variable ".\\RT Variables.lvlib\\Set1 full"(1.0) -> ()  [unwired: 1 in, 1 out]
        n124 = Equal?(x=w345, y=100) -> (x = y?=w349:bool)
        n125 = Select(t=T1."peque-reset" ("Enum"), s=w349, f=T1."peque- home" ("Enum")) -> (s? t:f=w346:T1)
      }
      frame "peque-reset" {
        w351 = TRUE
        w354 = 0.0 ("f")
        n126 = Select(t=T1."normal" ("Enum"), s=w351, f=T1."peque-reset" ("Enum")) -> (s? t:f=w352:T1)
      }
    }
    n127 = Select(t=w102, s=w104, f=w103) -> (s? t:f=w105:dbl)
    n128 = Greater Or Equal To 0?(x=w105) -> (x >= 0?=w136:bool)
    n129 = Less Than 0?(x=w105) -> (x < 0?=w135:bool)
    n130 = xnode "Digital output (1 sample)"("A/DIO0 (Pin 11)"=w136) -> ()  [unwired: 1 in, 1 out]
    n131 = xnode "Digital output (1 sample) 2"("A/DIO1 (Pin 13)"=w135) -> ()  [unwired: 1 in, 1 out]
    n132 = Greater Or Equal To 0?(x=w108) -> (x >= 0?=w144:bool)
    n133 = Less Than 0?(x=w108) -> (x < 0?=w143:bool)
    n134 = Get Date/Time In Seconds() -> (seconds since 1Jan1904=w231:timestamp)
    n135 = call <vilib>:"Set Duty Cycle.vi"("Duty Cycle"=w176, "PWM Ref In"=w224) -> ("error out"=w223:errorcluster, "PWM Ref Out"=w219:T3)  [unwired: 7 in]
    n136 = xnode "Digital output (1 sample) 4"("A/DIO3 (Pin 17)"=w143) -> ()  [unwired: 1 in, 1 out]
    n137 = xnode "Digital output (1 sample) 3"("A/DIO2 (Pin 15)"=w144) -> ()  [unwired: 1 in, 1 out]
    n138 = local write "Reset Counter"(w171) -> ()
    n139 = local write "Reset Counter 2"(w169) -> ()
    n140 = call <vilib>:"Set Duty Cycle.vi"("Duty Cycle"=w181, "PWM Ref In"=w183) -> ("error out"=w222:errorcluster, "PWM Ref Out"=w228:T3)  [unwired: 7 in]
    n141 = Merge Errors(w222, w223) -> (w221:errorcluster)
    n142 = xnode "PWM 2"("Duty Cycle"="Duty Cycle 2", "Frequency [Hz]"=w159) -> ()  [unwired: 1 in, 1 out]
    n143 = xnode "PWM"("Duty Cycle"="Duty Cycle", "Frequency [Hz]"=w159) -> ()  [unwired: 1 in, 1 out]
    n144 = xnode "Analog input (1 sample) 3"() -> ("stallBlanco (A/AI1 (Pin 5))"=w155:dbl, "stallRojo (A/AI0 (Pin 3))"=w154:dbl)  [unwired: 1 in, 1 out]
    "stallBlanco (A/AI1 (Pin 5))" <- w155
    "stallRojo (A/AI0 (Pin 3))" <- w154
    n145 = Bundle(w112, w108, "Counter Value"=w162, "seconds since 1Jan1904"=w231, w145, w99, w97) -> (w201:T24)  [unwired: 1 in]
    n146 = shared-variable ".\\RT Variables.lvlib\\Stop RT Loops"() -> (w230:bool)  [unwired: 1 in, 1 out]
    n147 = xnode "Button"() -> ("Value"=w161:bool)  [unwired: 1 in, 1 out]
    n148 = shared-variable ".\\RT Variables.lvlib\\Data"(w201, error in=w221) -> (error out=w229:errorcluster)
    n149 = Greater?(x=w154, y=100.0) -> (0:w186:bool)
    n150 = Greater?(x=w155, y=100.0) -> (0:w187:bool)
    n151 = Or(x=w229, y=w230) -> (x .or. y?=w218:bool)
    n152 = Or(x=w187, y=w186) -> (x .or. y?=w188:bool)
    n153 = Or(x=w161, y=w188) -> (x .or. y?=w185:bool)
    n154 = Or(x=w218, y=w185) -> (x .or. y?=w217:bool)
  }
  n155 = while {
    shift-right: [w654] -> w57
    shift-left: w16 -> [w652]
    tunnel: [w653] -> w58
    tunnel: w6 -> [w651]
    shift-right: [w650] -> _
    shift-left: enum16{"Connect", "Send"}."Connect" ("Message states") -> [w655]
    stop <- w656 stop-if-true
    # "Data sending loop"
    n156 = case shown="\"Connect\"" w655 {
      tunnel: [w660 w675] -> w653
      tunnel: [w658 w673] -> w654
      tunnel: [w664 w676] -> w650
      tunnel: w652 -> [_ w682]
      tunnel: w651 -> [w661 w681]
      frame "Connect" {
        # "Attempts connection with the UI every 5 seconds, once successful, proceeds to Send state."
        n157 = Create Network Stream Writer Endpoint(5:5000 ("timeout in ms (-1)"), 7:4096 ("writer buffer size"), 8:w661, 9:T25 {"Double"=0.0, "dbl Scaled Value"=0.0, "Output"=0.0, "seconds since 1Jan1904"=timestamp(0 s since 1904-01-01), 0.0, 0.0, 0.0} ("Data"), 11:"data writer" ("writer name")) -> (0:w662:errorcluster, 3:w659:refnum<k21>)  [unwired: 2 in]
        n158 = case shown="Error" w662 {
          selector: w662 -> [w667 _]
          tunnel: [enum16{"Connect", "Send"}."Send" ("Message states") enum16{"Connect", "Send"}."Connect" ("Message states")] -> w664
          tunnel: [w667 errorcluster {"status"=FALSE, "code"=0, "source"=""} ("error IO")] -> w660
          tunnel: w659 -> [w669 _]
          tunnel: [w669 w670] -> w658
          frame No Error {
          }
          frame Error {
            w670 = refnum<k21> refnum  # writer endpoint
          }
        }
      }
      frame "Send" {
        # "Sends deterministic loop acquired data to the UI."
        n159 = shared-variable ".\\RT Variables.lvlib\\Data"(error in=w681) -> (w678:T25, error out=w680:errorcluster)
        n160 = Unbundle By Name(w680) -> ("code"=w679:i32)
        n161 = case shown="0, Default" w679 {
          tunnel: [w695 w697] -> w677
          tunnel: [w694 w696] -> w674
          tunnel: w682 -> [w693 w696]
          tunnel: w680 -> [w692 w697]
          tunnel: w678 -> [w691 _]
          frame 0, Default {
            n162 = shared-variable-write(w693, w692, w691) -> (w694:refnum<k21>, w695:errorcluster)  [unwired: 1 in, 1 out]
          }
          frame -2220 {
            n163 = Wait (ms)(milliseconds to wait=u32 10) -> ()  [unwired: 1 out]
          }
        }
        n164 = case shown="Error" w677 {
          selector: w677 -> [w685 w689]
          tunnel: [enum16{"Connect", "Send"}."Send" ("Message states") enum16{"Connect", "Send"}."Connect" ("Message states")] -> w676
          tunnel: [w685 errorcluster {"status"=FALSE, "code"=0, "source"=""} ("error IO")] -> w675
          tunnel: w674 -> [w683 w688]
          tunnel: [w683 w686] -> w673
          frame No Error {
          }
          frame Error {
            w686 = refnum<k21> refnum  # writer endpoint
            n165 = Destroy Stream Endpoint(8:w689, 11:w688) -> ()  [unwired: 1 out]
          }
        }
      }
    }
    n166 = shared-variable ".\\RT Variables.lvlib\\Stop RT Loops"() -> (w656:bool)  [unwired: 1 in, 1 out]
  }
  n167 = while {
    tunnel: [w702] -> w54
    shift-right: [w706] -> _
    shift-left: refnum<k21> refnum ("reader endpoint") -> [w704]
    shift-right: [w705] -> _
    shift-left: enum16{"Connect", "Receive"}."Connect" ("Message states") -> [w707]
    tunnel: w6 -> [w703]
    tunnel: w6 -> [w700]
    stop <- w701 stop-if-true
    # "Message loop"
    n168 = case shown="\"Receive\"" w707 {
      tunnel: [w714 w731] -> _
      tunnel: [w712 w743] -> w706
      tunnel: [w721 w740] -> w705
      tunnel: w704 -> [_ w739]
      tunnel: w703 -> [_ w742]
      tunnel: [FALSE ("Stop RT Loops") w741] -> w701
      tunnel: w700 -> [_ w736]
      tunnel: [_ w732] -> w699
      frame "Connect" {
        # "Attempts connection with the UI every 5 seconds, once successful, proceeds to Receive state."
        n169 = Bundle("", variant, variant) -> (w717:cluster{string, variant, variant})  [unwired: 1 in]
        n170 = Create Network Stream Reader Endpoint(5:5000 ("timeout in ms (-1)"), 7:4096 ("reader buffer size"), 9:w717, 11:"message reader" ("reader name")) -> (0:w716:errorcluster, 3:w711:refnum<k21>)  [unwired: 3 in]
        n171 = case shown="Error" w716 {
          selector: w716 -> [w726 _]
          tunnel: [enum16{"Connect", "Receive"}."Receive" ("Message states") enum16{"Connect", "Receive"}."Connect" ("Message states")] -> w721
          tunnel: [w725 errorcluster {"status"=FALSE, "code"=0, "source"=""} ("error IO")] -> w714
          tunnel: [w724 refnum<k21> refnum ("reader endpoint")] -> w712
          tunnel: w711 -> [w724 _]
          frame No Error {
            n172 = shared-variable ".\\RT Variables.lvlib\\2setpoint"(w724, error in=w726) -> (error out=w725:errorcluster)
          }
          frame Error {
          }
        }
      }
      frame "Receive" {
        # "Receives messages from the UI."
        n173 = shared-variable-read(w739, w742) -> (w738:refnum<k21>, w744:errorcluster, w735:cluster{string, variant, variant})  [unwired: 1 in, 1 out]
        n174 = Unbundle(w735) -> (w746:string, w745:variant, w737:variant)
        n175 = case shown="\"Update setpoint\"" w746 {
          tunnel: w745 -> [_ w767 w782 w788 w806]
          tunnel: w744 -> [w751 w769 w771 w787 w800]
          tunnel: [w750 w764 w778 w789 _] -> w731
          tunnel: [refnum<k21> refnum ("reader endpoint") refnum<k21> refnum ("reader endpoint") w777 w795 w804] -> w743
          tunnel: w738 -> [w749 w763 w777 w795 w804]
          tunnel: [w747 w766 FALSE ("Stop RT Loops") FALSE ("Stop RT Loops") FALSE ("Stop RT Loops")] -> w741
          tunnel: [enum16{"Connect", "Receive"}."Connect" ("Message states") enum16{"Connect", "Receive"}."Receive" ("Message states") enum16{"Connect", "Receive"}."Receive" ("Message states") enum16{"Connect", "Receive"}."Receive" ("Message states") enum16{"Connect", "Receive"}."Receive" ("Message states")] -> w740
          tunnel: w737 -> [_ w759 w770 w791 w799]
          tunnel: w736 -> [_ w758 _ _ _]
          tunnel: [w747 _ _ _ w797] -> w734
          tunnel: [_ _ _ _ w796] -> w733
          frame "Disconnect UI", Default {
            w747 = FALSE ("Stop RT Loops")
            n176 = Destroy Stream Endpoint(8:w751, 11:w749) -> (0:w750:errorcluster)
          }
          frame "Stop" {
            n177 = Variant To Data(error in=w758, type=TRUE ("Stop RT Loops"), Variant=w759) -> (data=w756:bool, error out=w760:errorcluster)
            n178 = Variant To Data(error in=w769, type=TRUE ("Stop RT Loops"), Variant=w767) -> (data=w766:bool, error out=w768:errorcluster)
            n179 = shared-variable ".\\RT Variables.lvlib\\Stop RT Loops"(w766, error in=w768) -> (error out=w754:errorcluster)
            n180 = shared-variable ".\\RT Variables.lvlib\\Stop RT Loops"(w756, error in=w760) -> (error out=w755:errorcluster)
            n181 = Merge Errors(w754, w755) -> (w753:errorcluster)
            n182 = Destroy Stream Endpoint(8:w753, 11:w763) -> (0:w764:errorcluster)
          }
          frame "Update setpoint" {
            n183 = Variant To Data(error in=w771, type=0.0, Variant=w782) -> (data=w780:dbl, error out=w779:errorcluster)
            n184 = Variant To Data(error in=w771, type=0.0, Variant=w770) -> (data=w773:dbl, error out=w772:errorcluster)
            n185 = shared-variable ".\\RT Variables.lvlib\\Setpoint"(w780, error in=w779) -> (error out=w778:errorcluster)
            n186 = shared-variable ".\\RT Variables.lvlib\\Setpoint2"(w773, error in=w772) -> ()  [unwired: 1 out]
          }
          frame "Vector Setpoints" {
            n187 = Variant To Data(error in=w787, type=dbl[][][] [], Variant=w788) -> (data=w785:dbl[][][])  [unwired: 1 out]
            "vectores" <- w785
            n188 = Variant To Data(error in=w787, type=0.0, Variant=w791) -> (data=w790:dbl)  [unwired: 1 out]
            n189 = shared-variable ".\\RT Variables.lvlib\\Tiempo"(w790) -> (error out=w789:errorcluster)  [unwired: 1 in]
            n190 = Index Array(array=w785) -> (element #1=w784:dbl[][], element #2=w783:dbl[][])  [unwired: 6 in]
            "subarray" <- w784
            "subarray 2" <- w783
            n191 = shared-variable "myRIO-1900\\Untitled Library 7.lvlib\\subarray 2"(w783) -> ()  [unwired: 1 in, 1 out]
            n192 = shared-variable "myRIO-1900\\Untitled Library 6.lvlib\\subarray"(w784) -> ()  [unwired: 1 in, 1 out]
          }
          frame "Homing" {
            n193 = Variant To Data(error in=w800, type=TRUE, Variant=w806) -> (data=w797:bool, error out=w796:errorcluster)
            n194 = Variant To Data(error in=w800, type=0.0, Variant=w799) -> (data=→"data":dbl)  [unwired: 1 out]
          }
        }
        n195 = shared-variable ".\\RT Variables.lvlib\\Homing"(w734, error in=w733) -> (error out=w732:errorcluster)
      }
    }
    n196 = case shown="No Error" w699 {
      selector: w699 -> [w708 w709]
      tunnel: [w708 w709] -> w702
      frame No Error {
        # "No action required."
      }
      frame Error {
        # "Stops RT in case of error."
        n197 = shared-variable ".\\RT Variables.lvlib\\Stop RT Loops"(TRUE ("Stop RT Loops")) -> ()  [unwired: 1 in, 1 out]
      }
    }
  }
  n198 = Destroy Stream Endpoint(8:w58, 11:w57) -> (0:w55:errorcluster)
  n199 = node-c288(w61) -> ()  [unwired: 1 out]
  n200 = case shown="Error" w50 {
    selector: w50 -> [w807 w808]
    tunnel: [w807 w808] -> w12
    frame No Error {
      # "No action required."
    }
    frame Error {
      # "Destroys Message network stream to stop Message loop, in case of error."
      n201 = shared-variable ".\\RT Variables.lvlib\\2setpoint"() -> (w809:refnum<k21>)  [unwired: 1 in, 1 out]
      n202 = Destroy Stream Endpoint(11:w809) -> ()  [unwired: 1 in, 1 out]
    }
  }
  n203 = call <vilib>:"Stop.vi"("error in (no error)"=w12, "Encoder Ref In"=w42) -> ("error out"=w43:errorcluster, "Encoder Ref Out"=w44:T10)  [unwired: 8 in]
  n204 = call <vilib>:"Stop.vi"("error in (no error)"=w12, "Encoder Ref In"=w11) -> ("error out"=w14:errorcluster, "Encoder Ref Out"=w15:T10)  [unwired: 8 in]
  n205 = call <vilib>:"Close.vi"("error in (no error)"=w43, "Encoder Ref In"=w44) -> ("error out"=w37:errorcluster)  [unwired: 9 in]
  n206 = call <vilib>:"Close.vi"("error in (no error)"=w14, "Encoder Ref In"=w15) -> ("error out"=w13:errorcluster)  [unwired: 9 in]
  n207 = call <vilib>:"Close.vi"("error in (no error)"=w37, "PWM Ref In"=w34) -> ("error out"=w36:errorcluster)  [unwired: 9 in]
  n208 = call <vilib>:"Close.vi"("error in (no error)"=w13, "PWM Ref In"=w10) -> ("error out"=w9:errorcluster)  [unwired: 9 in]
  n209 = Merge Errors(w55, w54, w36, w9) -> (w53:errorcluster)
  n210 = shared-variable "myRIO-1900\\Network Shared Variables.lvlib\\error IO"(w53) -> ()  [unwired: 1 in, 1 out]
